vi "Write SLSC Switch Info.vi"(10 "SLSC Switch Info":T1[](array[typedef]), 11 "SLSC Switch in":refnum<class "SLSC Switch.lvclass">) -> (3 "SLSC Switch out":refnum<class "SLSC Switch.lvclass">)   [LabVIEW 2015, in "SLSC Switch.lvclass"]
uses:
  SLSC Switch.lvclass
  Controls/SLSC Relay Info.ctl
  SLSC Switch.lvclass/SLSC Switch.ctl
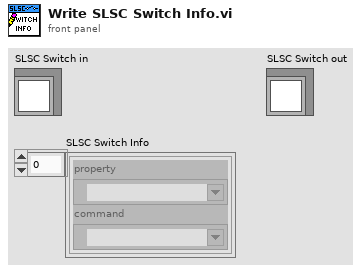
[diagram p1: front panel]
types:
  T1 = typedef "SLSC Switch.lvclass/SLSC Relay Info.ctl" = cluster{"property":refnum<k21>, "command":refnum<k21>}
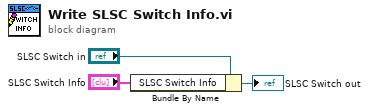
[diagram p0: block diagram]
diagram:
  n1 = Bundle By Name(cluster="SLSC Switch in", "SLSC Switch Info"="SLSC Switch Info") -> (→"SLSC Switch out":refnum<class "SLSC Switch.lvclass">)
